vi "例1_定长运动.vi"() -> ()   [LabVIEW 2012]
panel:
  in  "软件复位":bool
  in  "硬件复位":bool
  in  "总线状态":string
  in  "轴状态机":string
  in  "退出程序":bool
  in  "卡号":dbl
  in  "反馈位置 unit":dbl
  in  "当前位置 unit":dbl
  in  "当前速度 unit/s":dbl
  in  "指令清零":bool
  in  "设置脉冲当量":bool
  in  "停止运动":bool
  in  "执行运动":bool
  in  "在线变位":bool
  in  "目标位置 unit":dbl
  in  "在线变速":bool
  in  "变速时间 s":dbl
  in  "变速的运行速度 unit/s":dbl
  in  "运动状态":string
  in  "运动距离 unit":dbl
  in  "停止速度 unit/s":dbl
  in  "S段时间 s":dbl
  in  "减速时间 s":dbl
  in  "加速时间 s":dbl
  in  "运行速度 unit/s":dbl
  in  "起始速度 unit/s":dbl
  in  "脉冲当量  pulse/unit":dbl
  in  "电机轴号":dbl
  # "输入参数"
  # "在线变速"
  # "信息显示"
  # "在线变位"
  # "复位"
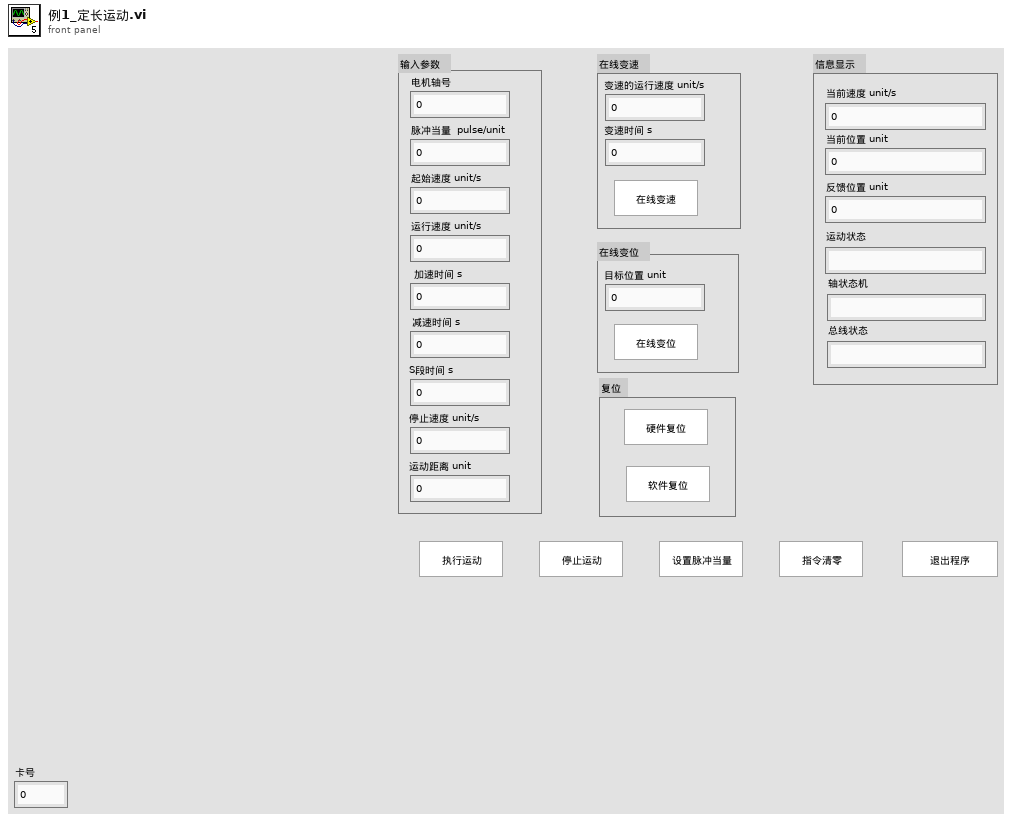
[diagram p1: front panel]
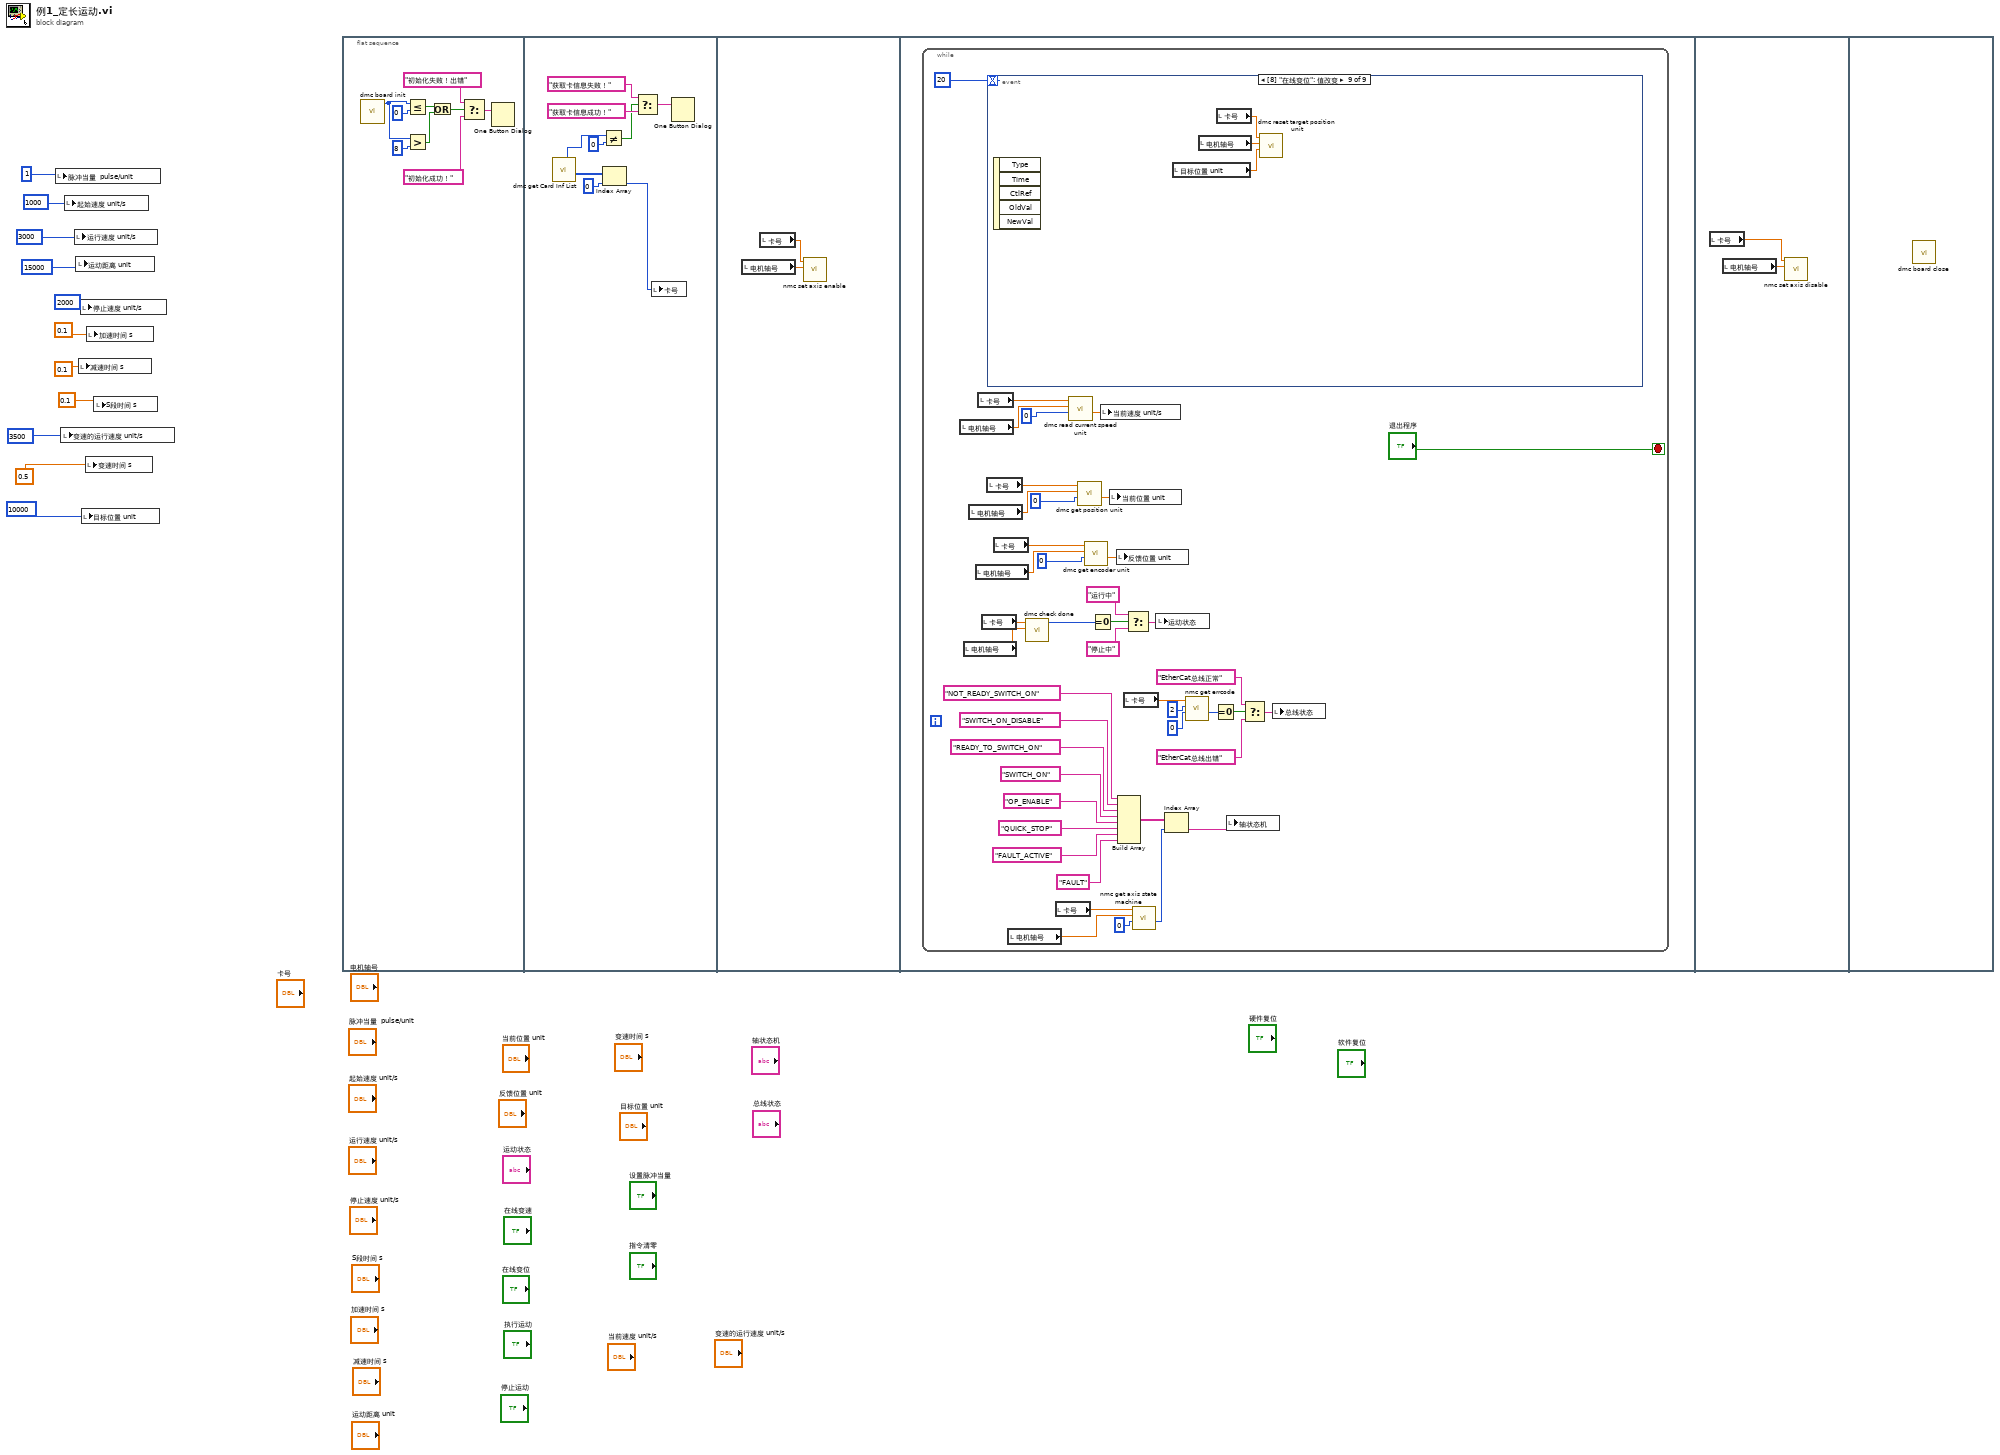
[diagram p0: block diagram]
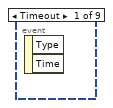
[diagram p2: hidden frame]
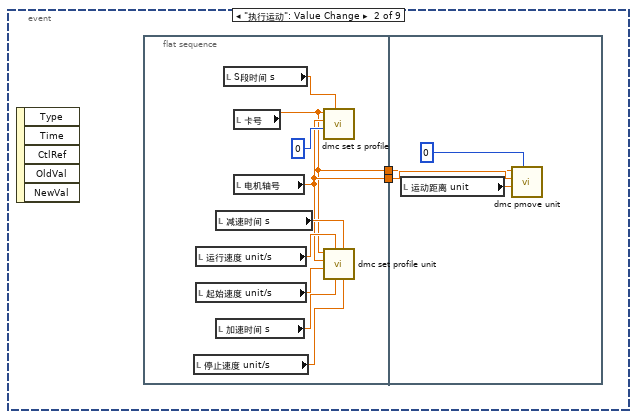
[diagram p3: hidden frame]
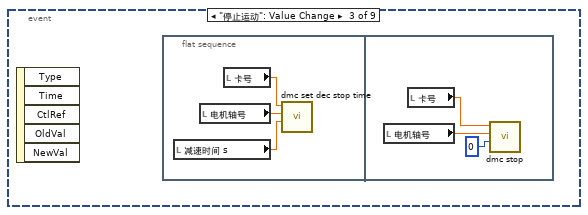
[diagram p4: hidden frame]
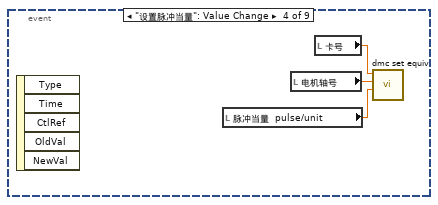
[diagram p5: hidden frame]
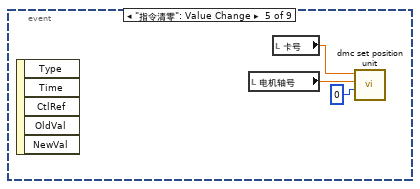
[diagram p6: hidden frame]
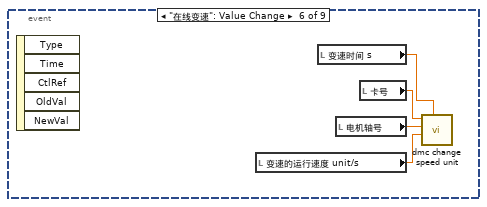
[diagram p7: hidden frame]
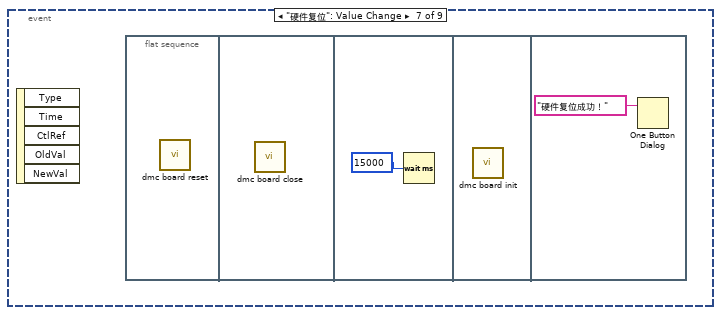
[diagram p8: hidden frame]
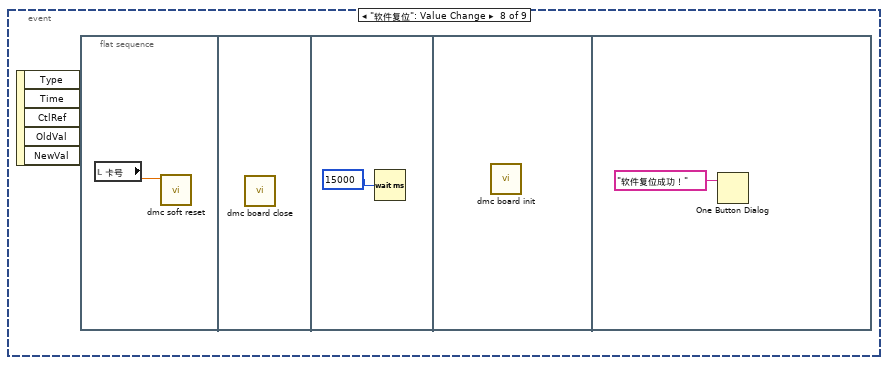
[diagram p9: hidden frame]
diagram:
  n1 = local write "脉冲当量  pulse/unit"(1) -> ()
  n2 = local write "变速的运行速度 unit/s"(3500) -> ()
  n3 = local write "起始速度 unit/s"(1000) -> ()
  n4 = local write "运行速度 unit/s"(3000) -> ()
  n5 = local write "运动距离 unit"(15000) -> ()
  n6 = local write "减速时间 s"(0.1) -> ()
  n7 = local write "停止速度 unit/s"(2000) -> ()
  n8 = local write "目标位置 unit"(10000) -> ()
  n9 = local write "变速时间 s"(0.5) -> ()
  n10 = local write "加速时间 s"(0.1) -> ()
  n11 = local write "S段时间 s"(0.1) -> ()
  n12 = flat-sequence {
    frame #0 {
      n13 = call "dmc board init.vi"() -> ("function return"=w13:i16)  [unwired: 10 in, 1 out]
      n14 = Less Or Equal?(x=w13, y=0) -> (x <= y?=w16:bool)
      n15 = Greater?(x=w13, y=8) -> (0:w15:bool)
      n16 = Or(x=w16, y=w15) -> (x .or. y?=w17:bool)
      n17 = Select(t="初始化失败！出错", s=w17, f="初始化成功！") -> (s? t:f=w19:string)
      n18 = One Button Dialog(message=w19) -> ()  [unwired: 1 in, 1 out]
    }
    frame #1 {
      n19 = call "dmc get Card Inf List.vi"() -> ("CardIdList out"=w23:u16[], "function return"=w24:i16)  [unwired: 7 in, 3 out]
      n20 = Not Equal?(x=w24, y=0) -> (x != y?=w26:bool)
      n21 = Index Array(array=w23, index=0) -> (element=w21:u16)
      n22 = Select(t="获取卡信息失败！", s=w26, f="获取卡信息成功！") -> (s? t:f=w29:string)
      n23 = local write "卡号"(w21) -> ()
      n24 = One Button Dialog(message=w29) -> ()  [unwired: 1 in, 1 out]
    }
    frame #2 {
      n25 = local read "电机轴号"() -> (w30:dbl)
      n26 = local read "卡号"() -> (w31:dbl)
      n27 = call "nmc set axis enable.vi"("axis"=w30, "CardNo"=w31) -> ()  [unwired: 8 in, 2 out]
    }
    frame #3 {
      n28 = while {
        stop <- "退出程序" stop-if-true
        n29 = local read "电机轴号"() -> (w59:dbl)
        n30 = local read "电机轴号"() -> (w60:dbl)
        n31 = local read "电机轴号"() -> (w69:dbl)
        n32 = local read "电机轴号"() -> (w67:dbl)
        n33 = local read "卡号"() -> (w58:dbl)
        n34 = local read "卡号"() -> (w55:dbl)
        n35 = local read "卡号"() -> (w57:dbl)
        n36 = event shown="[8] \"在线变位\": 值改变" {
          selector: _ -> [_ _ _ _ _ _ _ _ _]
          dyn-events: _ -> [_ _ _ _ _ _ _ _ _]
          timeout: 20 -> [_ _ _ _ _ _ _ _ _]
          event Timeout {
            n37 = event-data() -> ()  [unwired: 1 in, 2 out]
          }
          event "执行运动": Value Change {
            n38 = event-data() -> ()  [unwired: 1 in, 5 out]
            n39 = flat-sequence {
              tunnel: [w78] -> w76
              tunnel: [w77] -> w75
              tunnel: w76 -> [w87]
              tunnel: w75 -> [w86]
              frame #0 {
                n40 = local read "停止速度 unit/s"() -> (w85:dbl)
                n41 = local read "运行速度 unit/s"() -> (w82:dbl)
                n42 = local read "起始速度 unit/s"() -> (w81:dbl)
                n43 = local read "减速时间 s"() -> (w83:dbl)
                n44 = local read "加速时间 s"() -> (w84:dbl)
                n45 = local read "S段时间 s"() -> (w80:dbl)
                n46 = local read "卡号"() -> (w77:dbl)
                n47 = local read "电机轴号"() -> (w78:dbl)
                n48 = call "dmc set s profile.vi"("s_para"=w80, "s_mode"=0, "axis"=w78, "CardNo"=w77) -> ()  [unwired: 6 in, 2 out]
                n49 = call "dmc set profile unit.vi"("Stop_Vel"=w85, "Tdec"=w83, "Tacc"=w84, "Max_Vel"=w82, "Min_Vel"=w81, "axis"=w78, "CardNo"=w77) -> ()  [unwired: 3 in, 2 out]
              }
              frame #1 {
                n50 = local read "运动距离 unit"() -> (w88:dbl)
                n51 = call "dmc pmove unit.vi"("posi_mode"=0, "Dist"=w88, "axis"=w87, "CardNo"=w86) -> ()  [unwired: 6 in, 2 out]
              }
            }
          }
          event "停止运动": Value Change {
            n52 = event-data() -> ()  [unwired: 1 in, 5 out]
            n53 = flat-sequence {
              frame #0 {
                n54 = local read "减速时间 s"() -> (w91:dbl)
                n55 = local read "电机轴号"() -> (w92:dbl)
                n56 = local read "卡号"() -> (w90:dbl)
                n57 = call "dmc set dec stop time.vi"("time"=w91, "axis"=w92, "CardNo"=w90) -> ()  [unwired: 7 in, 2 out]
              }
              frame #1 {
                n58 = local read "电机轴号"() -> (w94:dbl)
                n59 = local read "卡号"() -> (w93:dbl)
                n60 = call "dmc stop.vi"("stop_mode"=0, "axis"=w94, "CardNo"=w93) -> ()  [unwired: 7 in, 2 out]
              }
            }
          }
          event "设置脉冲当量": Value Change {
            n61 = event-data() -> ()  [unwired: 1 in, 5 out]
            n62 = local read "脉冲当量  pulse/unit"() -> (w97:dbl)
            n63 = local read "电机轴号"() -> (w98:dbl)
            n64 = local read "卡号"() -> (w96:dbl)
            n65 = call "dmc set equiv.vi"("equiv"=w97, "axis"=w98, "CardNo"=w96) -> ()  [unwired: 7 in, 2 out]
          }
          event "指令清零": Value Change {
            n66 = event-data() -> ()  [unwired: 1 in, 5 out]
            n67 = local read "电机轴号"() -> (w101:dbl)
            n68 = local read "卡号"() -> (w99:dbl)
            n69 = call "dmc set position unit.vi"("pos"=0, "axis"=w101, "CardNo"=w99) -> ()  [unwired: 7 in, 2 out]
          }
          event "在线变速": Value Change {
            n70 = event-data() -> ()  [unwired: 1 in, 5 out]
            n71 = local read "变速的运行速度 unit/s"() -> (w103:dbl)
            n72 = local read "变速时间 s"() -> (w104:dbl)
            n73 = local read "电机轴号"() -> (w105:dbl)
            n74 = local read "卡号"() -> (w102:dbl)
            n75 = call "dmc change speed unit.vi"("Taccdec"=w104, "New_Vel"=w103, "axis"=w105, "CardNo"=w102) -> ()  [unwired: 6 in, 2 out]
          }
          event "硬件复位": Value Change {
            n76 = event-data() -> ()  [unwired: 1 in, 5 out]
            n77 = flat-sequence {
              frame #0 {
                n78 = call "dmc board reset.vi"() -> ()  [unwired: 10 in, 2 out]
              }
              frame #1 {
                n79 = call "dmc board close.vi"() -> ()  [unwired: 10 in, 2 out]
              }
              frame #2 {
                n80 = Wait (ms)(milliseconds to wait=15000) -> ()  [unwired: 1 out]
              }
              frame #3 {
                n81 = call "dmc board init.vi"() -> ()  [unwired: 10 in, 2 out]
              }
              frame #4 {
                n82 = One Button Dialog(message="硬件复位成功！") -> ()  [unwired: 1 in, 1 out]
              }
            }
          }
          event "软件复位": Value Change {
            n83 = event-data() -> ()  [unwired: 1 in, 5 out]
            n84 = flat-sequence {
              frame #0 {
                n85 = local read "卡号"() -> (w108:dbl)
                n86 = call "dmc soft reset.vi"("CardNo"=w108) -> ()  [unwired: 9 in, 2 out]
              }
              frame #1 {
                n87 = call "dmc board close.vi"() -> ()  [unwired: 10 in, 2 out]
              }
              frame #2 {
                n88 = Wait (ms)(milliseconds to wait=15000) -> ()  [unwired: 1 out]
              }
              frame #3 {
                n89 = call "dmc board init.vi"() -> ()  [unwired: 10 in, 2 out]
              }
              frame #4 {
                n90 = One Button Dialog(message="软件复位成功！") -> ()  [unwired: 1 in, 1 out]
              }
            }
          }
          event "在线变位": Value Change {
            n91 = event-data() -> ()  [unwired: 1 in, 5 out]
            n92 = local read "目标位置 unit"() -> (w112:dbl)
            n93 = local read "电机轴号"() -> (w113:dbl)
            n94 = local read "卡号"() -> (w111:dbl)
            n95 = call "dmc reset target position unit.vi"("New_Pos"=w112, "axis"=w113, "CardNo"=w111) -> ()  [unwired: 7 in, 2 out]
          }
        }
        n96 = local read "卡号"() -> (w56:dbl)
        n97 = local read "电机轴号"() -> (w52:dbl)
        n98 = call "dmc check done.vi"("axis"=w60, "CardNo"=w55) -> ("function return"=w61:i16)  [unwired: 8 in, 1 out]
        n99 = local read "卡号"() -> (w53:dbl)
        n100 = call "dmc read current speed unit.vi"("current_speed"=0, "axis"=w59, "CardNo"=w58) -> ("current_speed out"=w72:dbl)  [unwired: 6 in, 2 out]
        n101 = call "dmc get position unit.vi"("pos"=0, "axis"=w69, "CardNo"=w57) -> ("pos out"=w71:dbl)  [unwired: 6 in, 2 out]
        n102 = call "dmc get encoder unit.vi"("pos"=0, "axis"=w67, "CardNo"=w56) -> ("pos out"=w68:dbl)  [unwired: 6 in, 2 out]
        n103 = Equal To 0?(x=w61) -> (x = 0?=w64:bool)
        n104 = local write "当前速度 unit/s"(w72) -> ()
        n105 = local write "当前位置 unit"(w71) -> ()
        n106 = local write "反馈位置 unit"(w68) -> ()
        n107 = Build Array("NOT_READY_SWITCH_ON", "SWITCH_ON_DISABLE", "READY_TO_SWITCH_ON", "SWITCH_ON", "OP_ENABLE", "QUICK_STOP", "FAULT_ACTIVE", "FAULT") -> (w41:string[])
        n108 = local read "卡号"() -> (w40:dbl)
        n109 = Select(t="运行中" ("当前状态"), s=w64, f="停止中" ("当前状态")) -> (s? t:f=w65:string)
        n110 = call "nmc get axis state machine.vi"("Axis_StateMachine"=0, "axis"=w52, "CardNo"=w53) -> ("Axis_StateMachine out"=w50:u16)  [unwired: 6 in, 2 out]
        n111 = local write "运动状态"(w65) -> ()
        n112 = Index Array(array=w41, index=w50) -> (element=w32:string)
        n113 = call "nmc get errcode.vi"("Errcode"=0, "channel"=2, "CardNo"=w40) -> ("Errcode out"=w37:u16)  [unwired: 6 in, 2 out]
        n114 = Equal To 0?(x=w37) -> (x = 0?=w36:bool)
        n115 = local write "轴状态机"(w32) -> ()
        n116 = Select(t="EtherCat总线正常" ("当前状态"), s=w36, f="EtherCat总线出错" ("当前状态")) -> (s? t:f=w33:string)
        n117 = local write "总线状态"(w33) -> ()
      }
    }
    frame #4 {
      n118 = local read "卡号"() -> (w115:dbl)
      n119 = local read "电机轴号"() -> (w114:dbl)
      n120 = call "nmc set axis disable.vi"("axis"=w114, "CardNo"=w115) -> ()  [unwired: 8 in, 2 out]
    }
    frame #5 {
      n121 = call "dmc board close.vi"() -> ()  [unwired: 10 in, 2 out]
    }
  }
